vi "SwerveDrive.vi"() -> ()   [LabVIEW 2016]
uses:
  Refname/Motors.ctl
  Refname/Refname to String (Motors).vi
panel:
  in  "Y":dbl
  in  "X":dbl
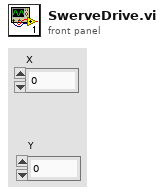
[diagram p1: front panel]
types:
  T1 = typedef "Motors.ctl" = enum16{"Wheel 1", "Swerve 1", "Wheel 2", "Swerve 2", "Wheel 3", "Swerve 3", "Wheel 4", "Swerve 4"}
  T2 = typedef "WPI_MotorControlDeviceRef.ctl" = cluster{"DeviceStatus":errorcluster, "Type":T3, "PWM":cluster{"PWM Channel":T4, "DeadBand":T5}, "CAN":cluster{"Device Number":u8, "SetOutput VI Ref":variant, "GetOutput VI Ref":variant, "Enable VI Ref":variant, "Disable VI Ref":variant, "Data":variant}, "Invert":bool}
  T3 = typedef "WPI_MotorControlType.ctl" = enum16{"PWM", "CAN"}
  T4 = typedef "FPGA_DIOPWMChannel.ctl" = enum8{"PWM 0", "PWM 1", "PWM 2", "PWM 3", "PWM 4", "PWM 5", "PWM 6", "PWM 7", "PWM 8", "PWM 9", "PWM MXP 0", "PWM MXP 1", "PWM MXP 2", "PWM MXP 3", "PWM MXP 4", "PWM MXP 5", "PWM MXP 6", "PWM MXP 7", "PWM MXP 8", "PWM MXP 9", "Invalid"}
  T5 = typedef "WPI_PWMDeadband.ctl" = cluster{"Name":string, "maxPositivePwm":i32, "minPositivePwm":i32, "centerPwm":i32, "maxNegativePwm":i32, "minNegativePwm":i32, "angularRange":u16}
  T6 = typedef "WPI_CANTalonSRX_GlobalStatus.ctl" = cluster{"Applied Throttle":dbl, "Module Enabled":bool, "CAN Error":errorcluster, "Closed Loop Error":dbl, "Forward Limit Switch Closed":bool, "Reverse Limit Switch Closed":bool, "Sensor Position":dbl, "Sensor Velocity":dbl, "Current":dbl, "Sticky Fault - Over Temp":bool, "Sticky Fault - Under Voltage":bool, "Sticky Fault - Forward Limit":bool, "Sticky Fault - Reverse Limit":bool, "Sticky Fault - Forward Soft Limit":bool, "Sticky Fault - Reverse Soft Limit":bool, "Brake is Enabled":bool, "Encoder Position":dbl, "Encoder Velocity":dbl, "Encoder Index Count":dbl, "Encoder A Pin State":bool, "Encoder B Pin State":bool, "Encoder Index Pin State":bool, "Analog In":dbl, "Analog In Velocity":dbl, "Temperature (C)":dbl, "Battery Voltage":dbl, "Control 5 Is Supported":bool, "Current Profile Slot Select":dbl, "Pos Div 8":bool, "Vel Div 4":bool, "Pulse Width Position":i32, "Pulse Width Velocity":i32, "Pulse Width Rise To Rise (us)":i32, "Pulse Width Rise To Fall (us)":i32, "Mot Prof Active Is Under Run":bool, "Mot Prof Active Has Under Run":bool, "Mot Prof Active Is Last":bool, "Mot Prof Active Velocity Only":bool, "Mot Prof Active Is Valid":bool, "Mot Prof Buffer Is Full":bool, "Mot Prof Active Profile Slot Select":i32, "Mot Prof NextID":i32, "Mot Prof Count":i32, "Mot Prof Active Velocity":dbl, "Mot Prof Active Position":dbl, "Mot Prof Output Enable":i32}
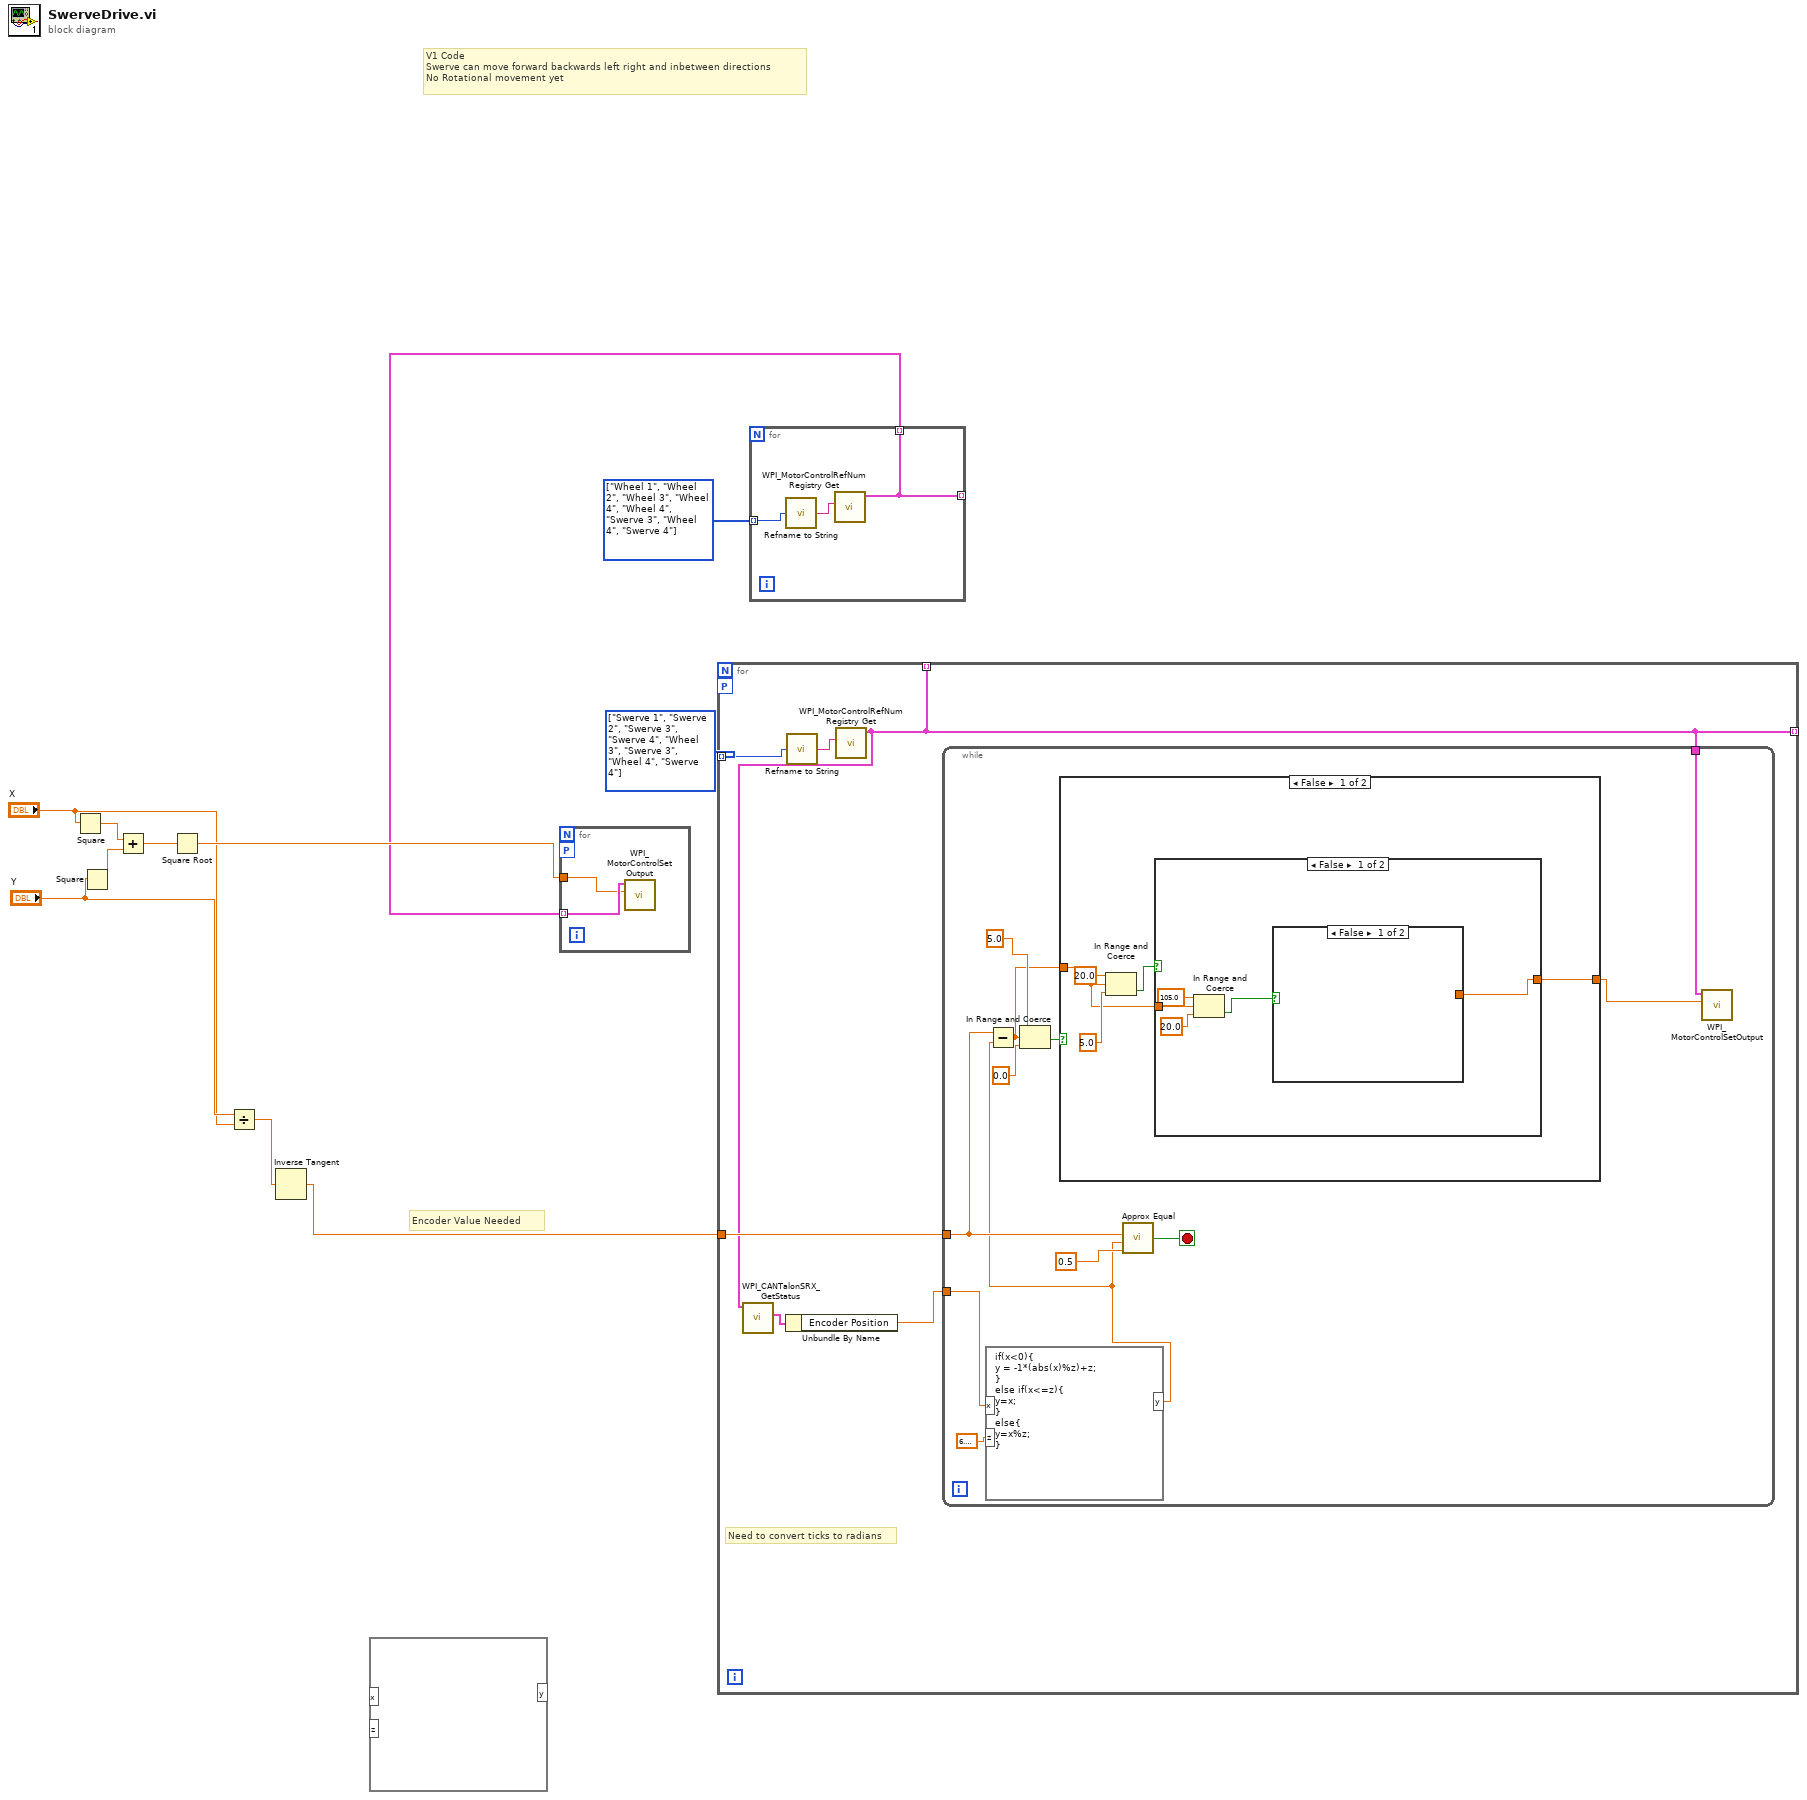
[diagram p0: block diagram]
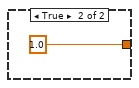
[diagram p2: hidden frame]
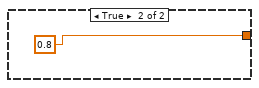
[diagram p3: hidden frame]
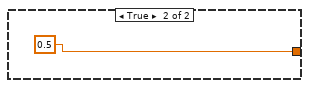
[diagram p4: hidden frame]
diagram:
  w10 = T1[] [enum."Swerve 1", enum."Swerve 2", enum."Swerve 3", enum."Swerve 4", enum."Wheel 3", enum."Swerve 3", enum."Wheel 4", enum."Swerve 4"] items=["Wheel 1", "Swerve 1", "Wheel 2", "Swerve 2", "Wheel 3", "Swerve 3", "Wheel 4", "Swerve 4"]
  w11 = T1[] [enum."Wheel 1", enum."Wheel 2", enum."Wheel 3", enum."Wheel 4", enum."Wheel 4", enum."Swerve 3", enum."Wheel 4", enum."Swerve 4"] items=["Wheel 1", "Swerve 1", "Wheel 2", "Swerve 2", "Wheel 3", "Swerve 3", "Wheel 4", "Swerve 4"]
  # "Encoder Value Needed"
  # "V1 Code\nSwerve can move forward backwards left right and inbetween directions\nNo Rotational movement yet"
  n1 = Square(x="X") -> (x^2=w7:dbl)
  n2 = Square(x="Y") -> (x^2=w8:dbl)
  n3 = Add(x=w7, y=w8) -> (x+y=w9:dbl)
  n4 = Square Root(x=w9) -> (sqrt(x)=w6:dbl)
  n5 = Divide(x="Y", y="X") -> (x/y=w3:dbl)
  n6 = Inverse Tangent(1:w3) -> (0:w1:dbl)
  n7 = formula code=""() -> ()  [unwired: 2 in, 1 out]
  n8 = for {
    tunnel: w10 -> [w17] mode=indexing
    tunnel: [w13] -> _ mode=indexing
    tunnel: [w13] -> _ mode=indexing
    workers-P: _ -> [_]
    tunnel: w1 -> [w14]
    # "Need to convert ticks to radians"
    n9 = call-poly "Refname to String.vi"("Enum"=w17) -> ("String"=w16:string)
    n10 = call <vilib>:"WPI_MotorControlRefNum Registry Get.vi"("refnum name"=w16) -> ("MotorControlDevRef"=w13:T2)  [unwired: 9 in, 1 out]
    n11 = call <vilib>:"WPI_CANTalonSRX_GetStatus.vi"("CAN Talon SRX Ref"=w13) -> ("Talon SRX Status"=w15:T6)  [unwired: 8 in, 2 out]
    n12 = Unbundle By Name(w15) -> ("Encoder Position"=w12:dbl)
    n13 = while {
      tunnel: w12 -> [w20]
      tunnel: w14 -> [w22]
      tunnel: w13 -> [w21]
      stop <- w28 stop-if-true
      n14 = formula code="if(x<0){\ny = -1*(abs(x)%z)+z;\n}\nelse if(x<=z){\ny=x;\n}\nelse{ \ny=x%z;\n}"("x"=w20, "z"=6.283185307179586) -> ("y"=w19:dbl)
      n15 = Subtract(x=w22, y=w19) -> (x-y=w24:dbl)
      n16 = In Range and Coerce(upper limit=5.0, x=w24, lower limit=0.0) -> (In Range?=w27:bool)  [unwired: 1 out]
      n17 = case shown="False" w27 {
        tunnel: w24 -> [w31 _]
        tunnel: [w30 0.5] -> w23
        frame False {
          n18 = In Range and Coerce(upper limit=20.0, x=w31, lower limit=5.0) -> (In Range?=w32:bool)  [unwired: 1 out]
          n19 = case shown="False" w32 {
            tunnel: w31 -> [w39 _]
            tunnel: [w35 0.8] -> w30
            frame False {
              n20 = In Range and Coerce(upper limit=105.0, x=w39, lower limit=20.0) -> (In Range?=w36:bool)  [unwired: 1 out]
              n21 = case shown="False" w36 {
                tunnel: [_ 1.0] -> w35
                frame False {
                }
                frame True {
                }
              }
            }
            frame True {
            }
          }
        }
        frame True {
        }
      }
      n22 = call "Approx Equal.vi"("Tolerance"=0.5, "b"=w19, "a"=w22) -> ("a == b?"=w28:bool)  [unwired: 1 in]
      n23 = call <vilib>:"WPI_MotorControlSetOutput.vi"("Output"=w23, "MotorControlDevRef"=w21) -> ()  [unwired: 7 in, 3 out]
    }
  }
  n24 = for {
    tunnel: w11 -> [w45] mode=indexing
    tunnel: [w43] -> _ mode=indexing
    tunnel: [w43] -> w2 mode=indexing
    n25 = call-poly "Refname to String.vi"("Enum"=w45) -> ("String"=w44:string)
    n26 = call <vilib>:"WPI_MotorControlRefNum Registry Get.vi"("refnum name"=w44) -> ("MotorControlDevRef"=w43:T2)  [unwired: 9 in, 1 out]
  }
  n27 = for {
    tunnel: w2 -> [w47] mode=indexing
    tunnel: w6 -> [w46]
    workers-P: _ -> [_]
    n28 = call <vilib>:"WPI_MotorControlSetOutput.vi"("Output"=w46, "MotorControlDevRef"=w47) -> ()  [unwired: 7 in, 3 out]
  }
